vi "Untitled 3.vi"   [LabVIEW 2020, in "CMESAPI.lvlib"]
uses:
  Libraries/CMESAPI/CMESAPI.lvlib
  Libraries/CMESAPI/CMESAPI.lvclass
panel:
  # "物品的睡觉哦靠"
  # "我的时间"
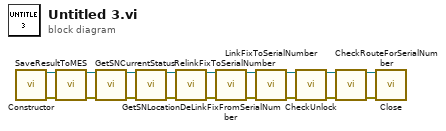
[diagram p0: block diagram]
diagram:
  n1 = call "Constructor.vi"() -> ("class data out"=w18:refnum<class "CMESAPI.lvclass">, "error out"=w17:errorcluster)  [unwired: 14 in]
  n2 = call-dynamic "SaveResultToMES.vi"("class data in"=w18, "error in (no error)"=w17) -> ("class data out"=w16:refnum<class "CMESAPI.lvclass">, "error out"=w15:errorcluster)  [unwired: 11 in, 1 out]
  n3 = call-dynamic "GetSNCurrentStatus.vi"("class data in"=w16, "error in (no error)"=w15) -> ("class data out"=w14:refnum<class "CMESAPI.lvclass">, "error out"=w13:errorcluster)  [unwired: 11 in, 1 out]
  n4 = call-dynamic "GetSNLocation.vi"("class data in"=w14, "error in (no error)"=w13) -> ("class data out"=w12:refnum<class "CMESAPI.lvclass">, "error out"=w11:errorcluster)  [unwired: 11 in, 1 out]
  n5 = call-dynamic "RelinkFixToSerialNumber.vi"("class data in"=w12, "error in (no error)"=w11) -> ("class data out"=w10:refnum<class "CMESAPI.lvclass">, "error out"=w9:errorcluster)  [unwired: 12 in]
  n6 = call-dynamic "DeLinkFixFromSerialNumber.vi"("class data in"=w10, "error in (no error)"=w9) -> ("class data out"=w8:refnum<class "CMESAPI.lvclass">, "error out"=w7:errorcluster)  [unwired: 11 in, 1 out]
  n7 = call-dynamic "LinkFixToSerialNumber.vi"("class data in"=w8, "error in (no error)"=w7) -> ("class data out"=w6:refnum<class "CMESAPI.lvclass">, "error out"=w5:errorcluster)  [unwired: 12 in]
  n8 = call-dynamic "CheckUnlock.vi"("class data in"=w6, "error in (no error)"=w5) -> ("class data out"=w4:refnum<class "CMESAPI.lvclass">, "error out"=w3:errorcluster)  [unwired: 11 in, 1 out]
  n9 = call-dynamic "CheckRouteForSerialNumber.vi"("class data in"=w4, "error in (no error)"=w3) -> ("class data out"=w2:refnum<class "CMESAPI.lvclass">, "error out"=w1:errorcluster)  [unwired: 11 in, 1 out]
  n10 = call-dynamic "Close.vi"("class data in"=w2, "error in (no error)"=w1) -> ()  [unwired: 13 in, 1 out]
